vi "TaskFor_OperatorLog_Message.vi"(8 "error in (no error)":errorcluster caption="错误输入（无错误）", 10 "事件文本":string, 11 "Input Operator输入":refnum<class "ControlPanel.lvclass">) -> (0 "error out":errorcluster caption="错误输出", 3 "Input Operator输出":refnum<class "ControlPanel.lvclass">)   [LabVIEW 2014, in "ControlPanel.lvlib" / "ControlPanel.lvclass"]
uses:
  ControlPanel.lvclass
  ControlPanel.lvclass/ControlPanel.ctl
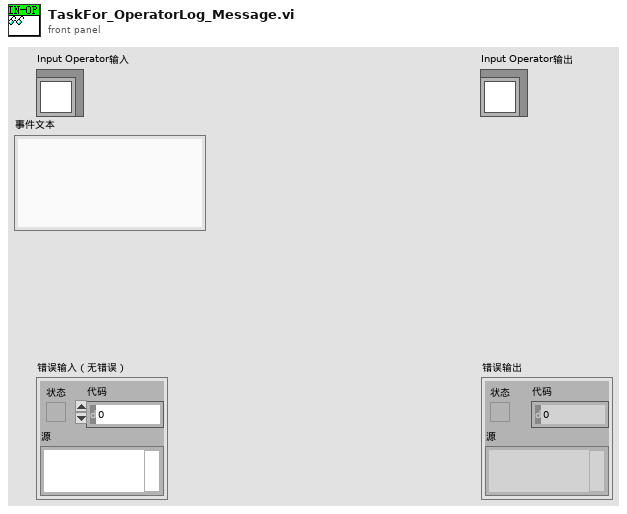
[diagram p1: front panel]
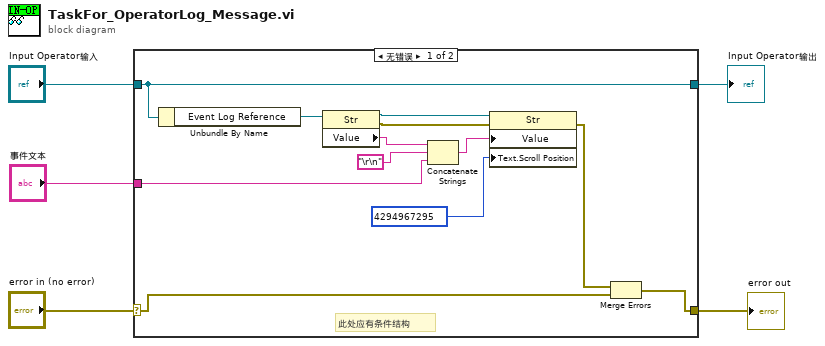
[diagram p0: block diagram]
diagram:
  n1 = case shown="无错误" "error in (no error)" {
    selector: "error in (no error)" -> [w8 w18]
    tunnel: [w6 w18] -> w4
    tunnel: [w17 w19] -> w2
    tunnel: "Input Operator输入" -> [w17 w19]
    tunnel: "事件文本" -> [w9 _]
    frame No Error {
      # "此处应有条件结构"
      n2 = Unbundle By Name(w17) -> ("Event Log Reference"=w16:refnum<vi>)
      n3 = property class="Str"(reference=w16) -> (reference out=w13:refnum<vi>, error out=w12:errorcluster, "Value"=w11:string)  [unwired: 1 in]
      n4 = Concatenate Strings(w11, "\r\n", w9) -> (w14:string)
      n5 = property class="Str"(reference=w13, error in=w12, "Value"=w14, "Text.Scroll Position"=u32 4294967295) -> (error out=w7:errorcluster)  [unwired: 1 out]
      n6 = Merge Errors(w7, w8) -> (w6:errorcluster)
    }
    frame Error {
    }
  }
  "error out" <- w4
  "Input Operator输出" <- w2
